vi "2x_reg.vi"(2 "WR":bool, 3 "RD":bool, 4 "C":bool, 6 "R":bool, 7 "I":T2) -> (0 "O_2":T1, 1 "O_1":T1)   [LabVIEW 2013]
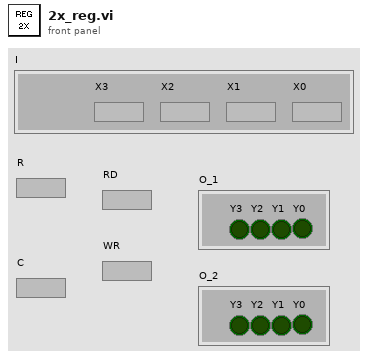
[diagram p1: front panel]
types:
  T1 = cluster{"Y3":bool, "Y2":bool, "Y1":bool, "Y0":bool}
  T2 = cluster{"X3":bool, "X2":bool, "X1":bool, "X0":bool}
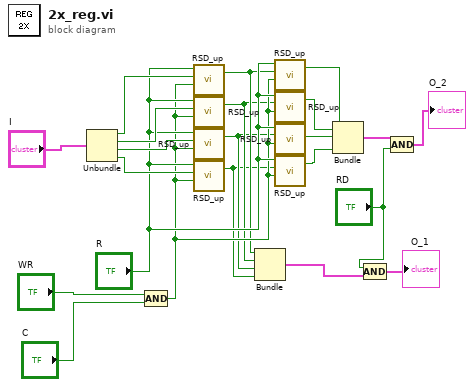
[diagram p0: block diagram]
diagram:
  n1 = Unbundle("I") -> ("X3"=w18:bool, "X2"=w17:bool, "X1"=w16:bool, "X0"=w15:bool)
  n2 = Compound Arithmetic op=AND("WR", "C") -> (w11:bool)
  n3 = call "RSD_up.vi"("C"=w11, "D"=w18, "R"="R") -> ("Q"=w7:bool)  [unwired: 1 in, 1 out]
  n4 = call "RSD_up.vi"("C"=w11, "D"=w17, "R"="R") -> ("Q"=w6:bool)  [unwired: 1 in, 1 out]
  n5 = call "RSD_up.vi"("C"=w11, "D"=w16, "R"="R") -> ("Q"=w5:bool)  [unwired: 1 in, 1 out]
  n6 = call "RSD_up.vi"("C"=w11, "D"=w15, "R"="R") -> ("Q"=w4:bool)  [unwired: 1 in, 1 out]
  n7 = Bundle("Q"=w7, "Q"=w6, "Q"=w5, "Q"=w4) -> (w2:cluster{"Q":bool, "Q":bool, "Q":bool, "Q":bool})  [unwired: 1 in]
  n8 = call "RSD_up.vi"("C"=w11, "D"=w7, "R"="R") -> ("Q"=w22:bool)  [unwired: 1 in, 1 out]
  n9 = call "RSD_up.vi"("C"=w11, "D"=w6, "R"="R") -> ("Q"=w21:bool)  [unwired: 1 in, 1 out]
  n10 = call "RSD_up.vi"("C"=w11, "D"=w5, "R"="R") -> ("Q"=w20:bool)  [unwired: 1 in, 1 out]
  n11 = call "RSD_up.vi"("C"=w11, "D"=w4, "R"="R") -> ("Q"=w19:bool)  [unwired: 1 in, 1 out]
  n12 = Bundle("Q"=w22, "Q"=w21, "Q"=w20, "Q"=w19) -> (w14:cluster{"Q":bool, "Q":bool, "Q":bool, "Q":bool})  [unwired: 1 in]
  n13 = Compound Arithmetic op=AND("RD", w2) -> (→"O_1":cluster{"Q":bool, "Q":bool, "Q":bool, "Q":bool})
  n14 = Compound Arithmetic op=AND(w14, "RD") -> (→"O_2":cluster{"Q":bool, "Q":bool, "Q":bool, "Q":bool})
